vi "SpreadsheetWrite.vi"(10 "input cluster":cluster{"Frequency":dbl[], "RMS":dbl[]}) -> ()   [LabVIEW 2014]
uses:
  <vilib>/Utility/file.llb/Write To Spreadsheet File (DBL).vi
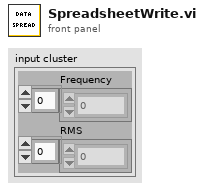
[diagram p1: front panel]
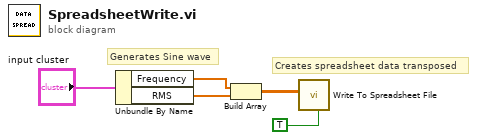
[diagram p0: block diagram]
diagram:
  # "Generates Sine wave"
  # "Creates spreadsheet data transposed"
  n1 = Unbundle By Name("input cluster") -> ("Frequency"=w4:dbl[], "RMS"=w3:dbl[])
  n2 = Build Array(w4, w3) -> (w2:dbl[][])
  n3 = call-poly <vilib>:"Write To Spreadsheet File.vi"("transpose? (no:F)"=TRUE, "2D data"=w2) -> ()  [unwired: 6 in, 1 out]
